vi "ManageAudioFiles.vi"(8 "error in (no error)":errorcluster, 11 "config":T1) -> (0 "error out":errorcluster, 3 "config out":T1)   [LabVIEW 2017, in "EmsaAudio.lvlib"]
uses:
  <vilib>/addons/InsightCM/Devices/Shared/Emsa/EmsaAudio/EmsaAudio.lvlib
  <vilib>/addons/InsightCM/Devices/Shared/Emsa/EmsaAudio/controls/config.ctl
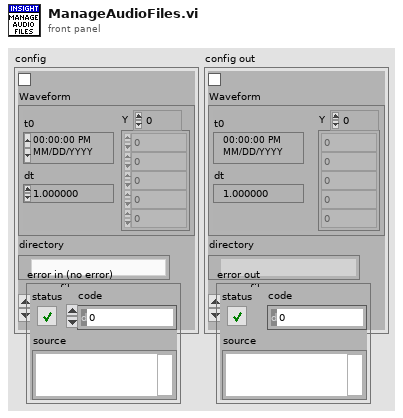
[diagram p1: front panel]
types:
  T1 = typedef "EmsaAudio.lvlib/config.ctl" = cluster{"Active":bool, "Waveform":waveform(dbl), "directory":path, "filenames":string[]}
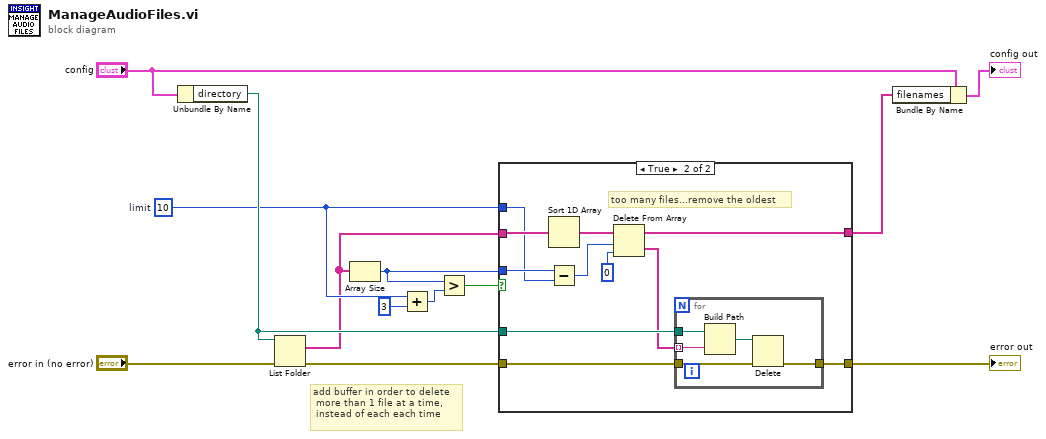
[diagram p0: block diagram]
diagram:
  w7 = 10  # limit
  # "add buffer in order to delete\n more than 1 file at a time,\n instead of each each time"
  n1 = Unbundle By Name("config") -> ("directory"=w8:path)
  n2 = List Folder(path=w8, error in="error in (no error)") -> (filenames=w6:string[], error out=w3:errorcluster)  [unwired: 2 in, 2 out]
  n3 = Array Size(array=w6) -> (size(s)=w5:i32)
  n4 = Add(x=w7, y=3) -> (x+y=w1:i32)
  n5 = Greater?(x=w5, y=w1) -> (0:w4:bool)
  n6 = case shown="True" w4 {
    tunnel: w3 -> [w15 w23]
    tunnel: w6 -> [w14 w26]
    tunnel: w5 -> [_ w25]
    tunnel: w7 -> [_ w24]
    tunnel: [w15 w22] -> w12
    tunnel: w8 -> [_ w21]
    tunnel: [w14 w16] -> w11
    frame False {
    }
    frame True {
      # "too many files...remove the oldest"
      n7 = Sort 1D Array(array=w26) -> (sorted array=w20:string[])
      n8 = Subtract(x=w25, y=w24) -> (x-y=w19:i32)
      n9 = Delete From Array(array=w20, length=w19, index=0) -> (deleted portion=w17:string[], array with subset deleted=w16:string[])
      n10 = for {
        tunnel: w23 -> [w31]
        tunnel: w17 -> [w27] mode=indexing
        tunnel: [w29] -> w22
        tunnel: w21 -> [w28]
        n11 = Build Path(base path=w28, name or relative path=w27) -> (appended path=w30:path)
        n12 = Delete(path (use dialog)=w30, error in=w31) -> (error out=w29:errorcluster)  [unwired: 3 in, 2 out]
      }
    }
  }
  "error out" <- w12
  n13 = Bundle By Name(cluster="config", "filenames"=w11) -> (→"config out":T1)
